vi "Generic command handler.vi"(8 "error in (no error)":errorcluster, 10 "Message in":refnum<class "GenericMessage.lvclass">, 11 "Piezo in":refnum<class "Piezo.lvclass">) -> (0 "error out":errorcluster, 2 "value":string, 3 "Piezo out":refnum<class "Piezo.lvclass">)   [LabVIEW 2012, in "Piezo.lvclass"]
doc: "The generic_command_handler processes the command 'generic'. Commands which are not part of the predefined list of commands fall under the 'generic' command for special activity."
uses:
  Piezo.lvclass
  <vilib>/Distrio/Murmex/GenericMessage/GenericMessage.lvclass
  <vilib>/Distrio/Murmex/Murmex/Murmex.lvclass
  Piezo.lvclass/Piezo.ctl
  <vilib>/DAQmx/write.llb/DAQmx Write (Analog DBL 1Chan 1Samp).vi
  <vilib>/Distrio/Murmex/Message/Message.lvclass
panel:
  # "This method is called when the GENERIC\ntrigger is sent. \n\nOverride this method when your component needs to\nrespond to this trigger. \n\nCall parent for proper implementation"
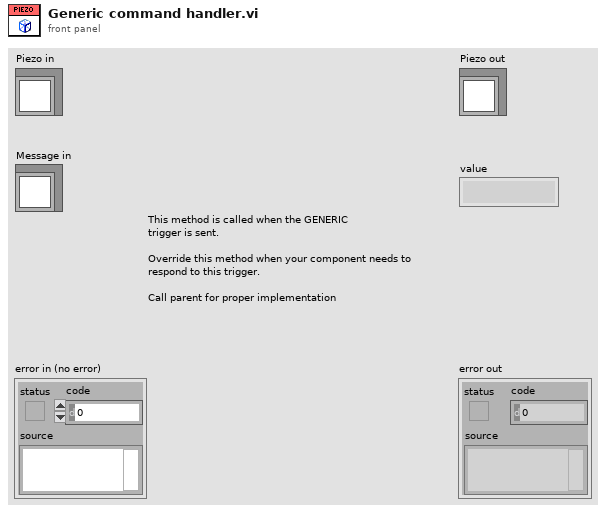
[diagram p1: front panel]
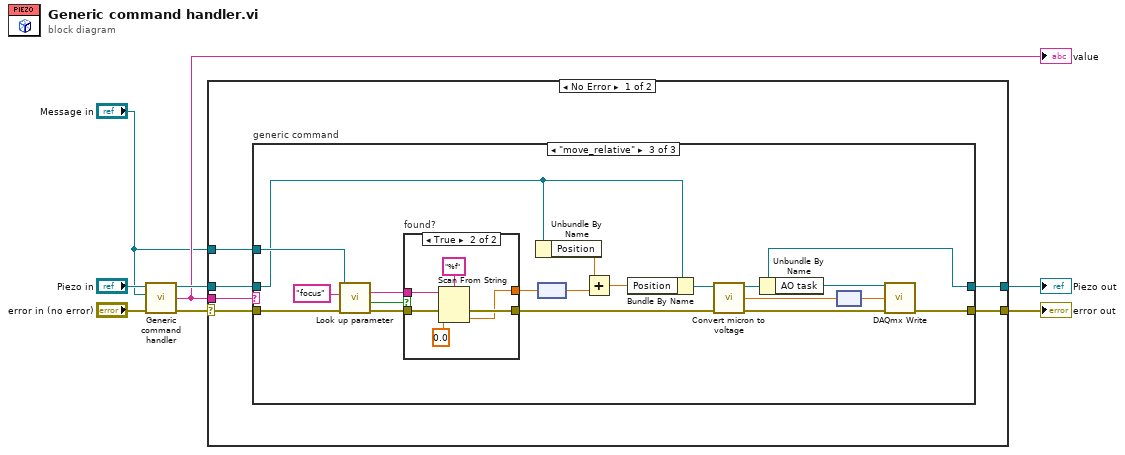
[diagram p0: block diagram]
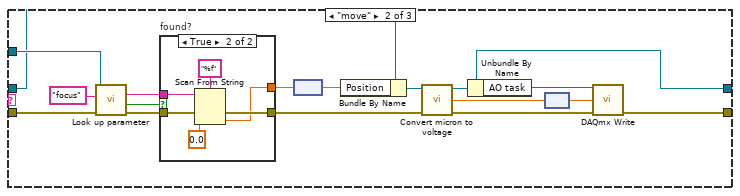
[diagram p3: hidden frame]
diagram:
  n1 = call-parent "Generic command handler.vi"("error in (no error)"="error in (no error)", "Message in"="Message in", "Murmex in"="Piezo in") -> ("error out"=w6:errorcluster, "value"=w2:string, "Murmex out"=w3:refnum<class "Piezo.lvclass">)  [unwired: 6 in]
  "value" <- w2
  n2 = case shown="No Error" w6 {
    selector: w6 -> [w12 w67]
    tunnel: w2 -> [w14 _]
    tunnel: [w13 w67] -> w5
    tunnel: [w11 w68] -> w4
    tunnel: w3 -> [w10 w68]
    tunnel: "Message in" -> [w9 _]
    frame No Error {
      n3 = case "generic command" shown="\"move_relative\"" w14 {
        tunnel: [w16 w21 w49] -> w13
        tunnel: w12 -> [w16 w32 w58]
        tunnel: [w15 w17 w45] -> w11
        tunnel: w10 -> [w15 w26 w44]
        tunnel: w9 -> [_ w33 w59]
        frame Default {
        }
        frame "move" {
          n4 = call <vilib>:"Look up parameter.vi"("error in (no error)"=w32, "name"="focus", "Message in"=w33) -> ("error out"=w29:errorcluster, "found?"=w30:bool, "key"=w28:string)  [unwired: 5 in, 1 out]
          n5 = case "found?" shown="True" w30 {
            tunnel: w29 -> [w34 w39]
            tunnel: w28 -> [_ w38]
            tunnel: [w34 w36] -> w23
            tunnel: [_ w35] -> w27
            frame False {
            }
            frame True {
              n6 = Scan From String(format string="%f", input string=w38, error in=w39, default 1=0.0 ("default value 1")) -> (error out=w36:errorcluster, output 1=w35:dbl)  [unwired: 1 in, 2 out]
            }
          }
          n7 = node(w27) -> (w25:dbl[unit])
          n8 = Bundle By Name(cluster=w26, "Position"=w25) -> (w24:refnum<class "Piezo.lvclass">)
          n9 = call-dynamic "Convert micron to voltage.vi"("error in (no error)"=w23, "Piezo in"=w24) -> ("error out"=w22:errorcluster, "Output voltage"=w19:dbl[unit], "Piezo out"=w17:refnum<class "Piezo.lvclass">)  [unwired: 7 in]
          n10 = Unbundle By Name(w17) -> ("AO task"=w20:refnum<k21>)
          n11 = node(w19) -> (w18:dbl)
          n12 = call-poly <vilib>:"DAQmx Write.vi"("task/channels in"=w20, "data"=w18, "error in"=w22) -> ("error out"=w21:errorcluster)  [unwired: 10 in, 2 out]
        }
        frame "move_relative" {
          n13 = call <vilib>:"Look up parameter.vi"("error in (no error)"=w58, "name"="focus", "Message in"=w59) -> ("error out"=w55:errorcluster, "found?"=w56:bool, "key"=w54:string)  [unwired: 5 in, 1 out]
          n14 = case "found?" shown="True" w56 {
            tunnel: w55 -> [w60 w65]
            tunnel: w54 -> [_ w64]
            tunnel: [w60 w62] -> w51
            tunnel: [_ w61] -> w53
            frame False {
            }
            frame True {
              n15 = Scan From String(format string="%f", input string=w64, error in=w65, default 1=0.0 ("default value 1")) -> (error out=w62:errorcluster, output 1=w61:dbl)  [unwired: 1 in, 2 out]
            }
          }
          n16 = Unbundle By Name(w44) -> ("Position"=w43:dbl[unit])
          n17 = node(w53) -> (w42:dbl[unit])
          n18 = Add(x=w43, y=w42) -> (x+y=w41:dbl[unit])
          n19 = Bundle By Name(cluster=w44, "Position"=w41) -> (w52:refnum<class "Piezo.lvclass">)
          n20 = call-dynamic "Convert micron to voltage.vi"("error in (no error)"=w51, "Piezo in"=w52) -> ("error out"=w50:errorcluster, "Output voltage"=w47:dbl[unit], "Piezo out"=w45:refnum<class "Piezo.lvclass">)  [unwired: 7 in]
          n21 = Unbundle By Name(w45) -> ("AO task"=w48:refnum<k21>)
          n22 = node(w47) -> (w46:dbl)
          n23 = call-poly <vilib>:"DAQmx Write.vi"("task/channels in"=w48, "data"=w46, "error in"=w50) -> ("error out"=w49:errorcluster)  [unwired: 10 in, 2 out]
        }
      }
    }
    frame Error {
    }
  }
  "error out" <- w5
  "Piezo out" <- w4
